vi "污染物CP编码.vi"(5 "-flag=":string="-Flag=", 7 "Type/标识":string="N", 8 "字段结束":bool=TRUE, 10 "污染物浓度":string[](array[string]), 11 "因子编码&数据类型":cluster{"因子编码":string, "数据类型":string}[](array[cluster])) -> (3 "编码输出":string)   [LabVIEW 2016, in "中水三立SQL数据传输.lvlib" / "HJ212.lvclass"]
uses:
  HJ212.lvclass
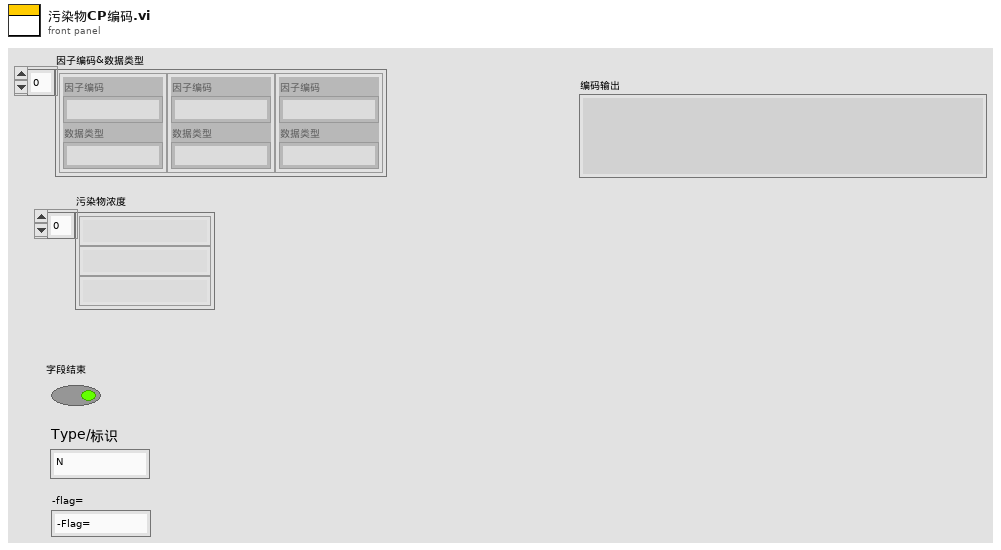
[diagram p1: front panel]
types:
  T1 = cluster{"因子编码":string, "数据类型":string, "污染物浓度":string}
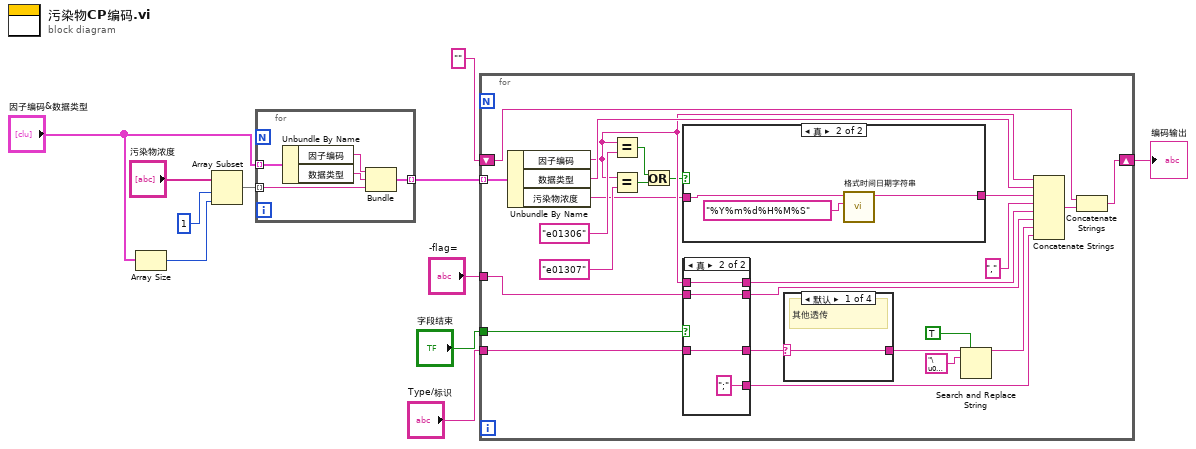
[diagram p0: block diagram]
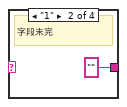
[diagram p3: hidden frame]
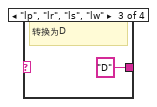
[diagram p4: hidden frame]
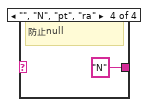
[diagram p5: hidden frame]
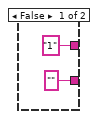
[diagram p6: hidden frame]
diagram:
  n1 = Array Size(array="因子编码&数据类型") -> (size(s)=w6:i32)
  n2 = Array Subset(array="污染物浓度", index=1 ("索引"), length=w6) -> (w5:string[])
  n3 = for {
    tunnel: "因子编码&数据类型" -> [w16] mode=indexing
    tunnel: w5 -> [w13] mode=indexing
    tunnel: [w12] -> w2 mode=indexing
    n4 = Unbundle By Name(w16) -> ("因子编码"=w15:string, "数据类型"=w14:string)
    n5 = Bundle("因子编码"=w15, "数据类型"=w14, "污染物浓度"=w13) -> (w12:T1)  [unwired: 1 in]
  }
  n6 = for {
    tunnel: "字段结束" -> [w39]
    tunnel: w2 -> [w26] mode=indexing
    tunnel: "Type/标识" -> [w30]
    tunnel: "-flag=" -> [w31]
    shift-right: [w27] -> w11
    shift-left: "" -> [w29]
    n7 = Unbundle By Name(w26) -> ("因子编码"=w20:string, "数据类型"=w25:string, "污染物浓度"=w17:string)
    n8 = Equal?(x=w20, y="e01306") -> (x = y?=w23:bool)
    n9 = Equal?(x=w20, y="e01307") -> (x = y?=w21:bool)
    n10 = Or(x=w23, y=w21) -> (x .or. y?=w19:bool)
    n11 = case shown="真" w19 {
      tunnel: w17 -> [w42 w45]
      tunnel: [w42 w43] -> w18
      frame False {
      }
      frame True {
        n12 = call "格式时间日期字符串.vi"("时间格式字符串(%c)"="%Y%m%d%H%M%S", "字符串"=w45) -> ("result string"=w43:string)  [unwired: 9 in]
      }
    }
    n13 = case shown="真" w39 {
      tunnel: [_ w53] -> w40
      tunnel: ["1" ("字符串") w52] -> w37
      tunnel: w20 -> [_ w55]
      tunnel: [_ w55] -> w38
      tunnel: ["" ("字符串") ";" ("字符串")] -> w32
      tunnel: w31 -> [_ w53]
      tunnel: w30 -> [_ w52]
      frame False {
      }
      frame True {
      }
    }
    n14 = case shown="默认" w37 {
      selector: w37 -> [w46 _ _ _]
      tunnel: [w46 "" ("字符串") "D" ("字符串") "N" ("字符串")] -> w36
      frame Default {
        # "其他透传"
      }
      frame "1" {
        # "字段未完"
      }
      frame "lp", "lr", "ls", "lw" {
        # "转换为D"
      }
      frame "", "N", "pt", "ra" {
        # "防止null"
      }
    }
    n15 = Search and Replace String(replace all?=TRUE ("替换全部？(F)"), input string=w36, search string="\u0000" ("搜索字符串")) -> (result string=w34:string)  [unwired: 5 in, 3 out]
    n16 = Concatenate Strings(w20, w25, w18, "," ("字符串"), w38, w40, w34, w32) -> (w28:string)
    n17 = Concatenate Strings(w29, w28) -> (w27:string)
  }
  "编码输出" <- w11
